vi "Test Call Inherited Test.vi"(8 "error in (no error)":errorcluster, 11 "Test Case In":refnum<class "Inheritance Test.lvclass">) -> (0 "error out":errorcluster, 3 "Test Case Out":refnum<class "Inheritance Test.lvclass">)   [LabVIEW 2020, in "Inheritance Test.lvclass"]
uses:
  Inheritance Test.lvclass
  C:/Program Files (x86)/National Instruments/LabVIEW 2020/vi.lib/Astemes/LUnit/Test Case.lvclass
  Test Doubles/Test Case Test Double/Test Case Test Double Child.lvclass
  Test Doubles/Test Case Test Double Parent/Test Case Test Double Parent.lvclass
  <vilib>/Astemes/LUnit/Test Case.lvclass/Test Case.ctl
  e8c5eeff-a694-4c0d-b261-74e2e6f5327d.vi
  <vilib>/Astemes/LUnit/Append Pass Result.vi
  <vilib>/Astemes/LUnit/Append Fail Result.vi
  <vilib>/Astemes/LUnit/Describe Comparison.vi
  <vilib>/Astemes/LUnit/Compare Variants.vi
  <vilib>/Astemes/LUnit/Run In UI.vi
  <vilib>/Utility/error.llb/Clear Errors.vi
  <vilib>/Utility/LVClass/Get LV Class Name.vi
  <vilib>/Astemes/LUnit/Describe Variant.vi
  Inheritance Test.lvclass/Inheritance Test.ctl
  <vilib>/Astemes/LUnit/Test Case.lvclass
  C:/git/astemes-lunit/source/API/LUnit Inheriting Test Case/LUnit Inheriting Test Case.lvclass
  C:/Program Files (x86)/National Instruments/LabVIEW 2020/vi.lib/Astemes/LUnit/LUnit Runnable.lvclass
  C:/git/astemes-lunit/tests/Test Doubles/Test Case Test Double Parent/Test Case Test Double Parent.lvclass
  C:/git/astemes-lunit/tests/Test Doubles/Test Case Test Double/Test Case Test Double Child.lvclass
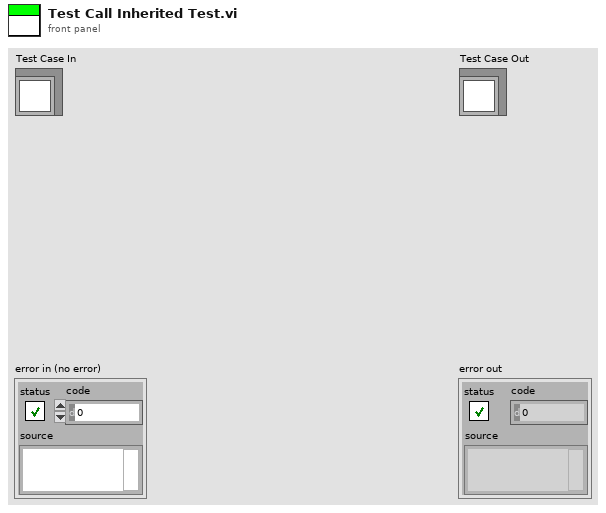
[diagram p1: front panel]
types:
  T1 = enum16{"", "Passed", "Failed", "Error", "Skipped", "Setup Error", "Broken", "Teardown Error"}
  T2 = cluster{"Name":string, "Message":string, "Description":string, "Status":enum16{"", "Passed", "Failed", "Error", "Skipped", "Setup Error", "Broken", "Teardown Error"}, "Result Type":enum16{"Test Case", "Test Suite", "Test Run", "Pass", "Fail", "Skip", "Pass if", "Fail if", "Pass if Error", "Fail if Error", "Pass if Equal", "Fail if Equal"}, "Execution Time":dbl}[]
  T3 = cluster{"Name":string, "Message":string, "Description":string, "Status":enum16{"", "Passed", "Failed", "Error", "Skipped", "Setup Error", "Broken", "Teardown Error"}, "Result Type":enum16{"Test Case", "Test Suite", "Test Run", "Pass", "Fail", "Skip", "Pass if", "Fail if", "Pass if Error", "Fail if Error", "Pass if Equal", "Fail if Equal"}, "Execution Time":dbl}
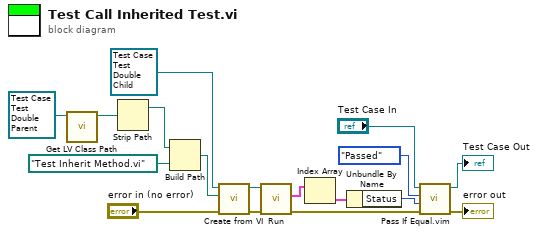
[diagram p0: block diagram]
diagram:
  n1 = call <vilib>:"Get LV Class Path.vi"("object"=refnum<class "Test Case Test Double Parent.lvclass"> refnum ("Test Case Test Double Parent.lvclass")) -> ("class path"=w5:path)  [unwired: 9 in, 1 out]
  n2 = Strip Path(path=w5) -> (stripped path=w6:path)  [unwired: 1 out]
  n3 = Build Path(base path=w6, name or relative path=path "Test Inherit Method.vi") -> (appended path=w1:path)
  n4 = call <vilib>:"Create from VI.vi"("error in (no error)"="error in (no error)", "Test Method VI Path"=w1, "LUnit Test Case Class"=refnum<class "Test Case Test Double Child.lvclass"> refnum ("LUnit Test Case V2 Test Double Child.lvclass")) -> ("error out"=w13:errorcluster, "LUnit Test Case Out"=w14:refnum<class "Test Case Test Double Child.lvclass">)  [unwired: 7 in]
  n5 = call-dynamic "Run.vi"("error in (no error)"=w13, "LUnit Inheriting Test Case In"=w14) -> ("error out"=w11:errorcluster, "Results"=w10:T2)  [unwired: 6 in, 2 out]
  n6 = Index Array(array=w10) -> (element=w9:T3)  [unwired: 1 in]
  n7 = Unbundle By Name(w9) -> ("Status"=w8:T1)
  n8 = call "Pass If Equal.vim"("error in (no error)"=w11, "Actual"=w8, "Expected"=T1."Passed" ("Status"), "LUnit Test Case In"="Test Case In") -> ("error out"=→"error out":errorcluster, "LUnit Test Case Out"=→"Test Case Out":refnum<class "Inheritance Test.lvclass">)  [unwired: 6 in]
